vi "Clear Display.vi"(6 "chip select  (1st chip)":enum16{"1st chip", "2nd chip"}(ring), 8 "error in (no error)":errorcluster, 11 "LCD in":refnum<class "Character LCD.lvclass">) -> (0 "error out":errorcluster, 3 "LCD out":refnum<class "Character LCD.lvclass">)   [LabVIEW 2015, in "HD44780 Host.lvlib"]
uses:
  HD44780 Host.lvlib
  Internal/LCD Class/Character LCD.lvclass
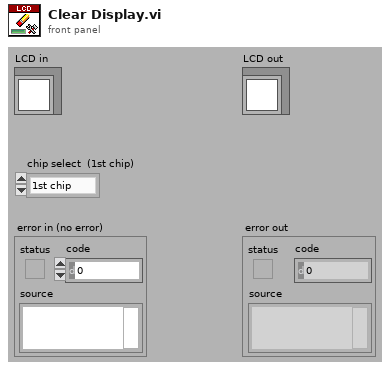
[diagram p1: front panel]
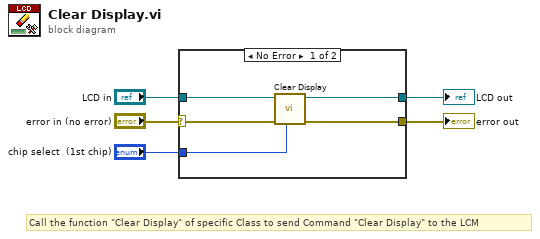
[diagram p0: block diagram]
diagram:
  # "Call the function \"Clear Display\" of specific Class to send Command \"Clear Display\" to the LCM"
  n1 = case shown="No Error" "error in (no error)" {
    selector: "error in (no error)" -> [w6 w12]
    tunnel: "chip select  (1st chip)" -> [w10 _]
    tunnel: [w8 w12] -> w3
    tunnel: "LCD in" -> [w9 w11]
    tunnel: [w7 w11] -> w1
    frame No Error {
      n2 = call-dynamic "Clear Display.vi"("chip select  (1st chip)"=w10, "error in (no error)"=w6, "Character LCD in"=w9) -> ("error out"=w8:errorcluster, "Character LCD out"=w7:refnum<class "Character LCD.lvclass">)  [unwired: 7 in]
    }
    frame Error {
    }
  }
  "error out" <- w3
  "LCD out" <- w1
